vi "Pos2Ins.vi"(1 "Pos":dbl) -> (0 "Ins":i32[](array[numeric]))   [LabVIEW 2016]
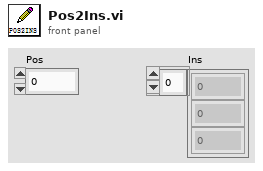
[diagram p1: front panel]
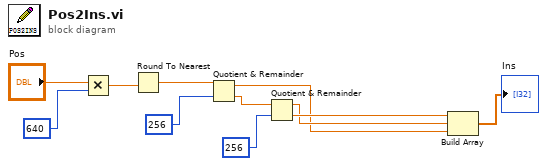
[diagram p0: block diagram]
diagram:
  n1 = Multiply(x="Pos", y=640) -> (x*y=w9:dbl)
  n2 = Round To Nearest(number=w9) -> (nearest integer value=w8:dbl)
  n3 = Quotient & Remainder(x=w8, y=256) -> (x-y*floor(x/y)=w2:dbl, floor(x/y)=w6:dbl)
  n4 = Quotient & Remainder(x=w6, y=256) -> (x-y*floor(x/y)=w3:dbl, floor(x/y)=w4:dbl)
  n5 = Build Array(w4, w3, w2) -> (→"Ins":dbl[])
